vi "get matrix.vi"(8 "error in":errorcluster {"code" format="%.0x"}, 10 "Output Subunit":u32=1, 11 "Input Handle":cluster{"Session":u32, "Card number":u32}) -> (0 "error out":errorcluster, 1 "第二行":T1, 2 "第一行":T1, 3 "Output Handle":cluster{"Session":u32, "Card number":u32})   [LabVIEW 2018]
uses:
  ctl/matrix.ctl
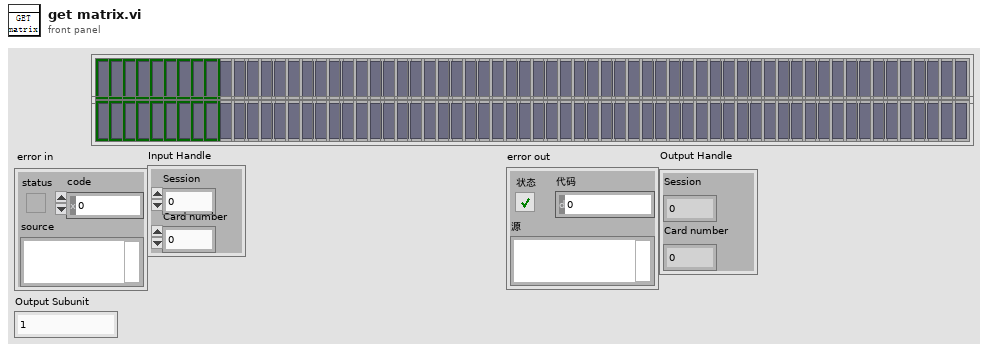
[diagram p1: front panel]
types:
  T1 = typedef "matrix.ctl" = cluster{"布尔":bool, "布尔 2":bool, "布尔 3":bool, "布尔 4":bool, "布尔 5":bool, "布尔 6":bool, "布尔 7":bool, "布尔 8":bool, "布尔 9":bool, "布尔 10":bool, "布尔 11":bool, "布尔 12":bool, "布尔 13":bool, "布尔 14":bool, "布尔 15":bool, "布尔 16":bool, "布尔 17":bool, "布尔 18":bool, "布尔 19":bool, "布尔 20":bool, "布尔 21":bool, "布尔 22":bool, "布尔 23":bool, "布尔 24":bool, "布尔 25":bool, "布尔 26":bool, "布尔 27":bool, "布尔 28":bool, "布尔 29":bool, "布尔 30":bool, "布尔 31":bool, "布尔 32":bool, "布尔 33":bool, "布尔 34":bool, "布尔 35":bool, "布尔 36":bool, "布尔 37":bool, "布尔 38":bool, "布尔 39":bool, "布尔 40":bool, "布尔 41":bool, "布尔 42":bool, "布尔 43":bool, "布尔 44":bool, "布尔 45":bool, "布尔 46":bool, "布尔 47":bool, "布尔 48":bool, "布尔 49":bool, "布尔 50":bool, "布尔 51":bool, "布尔 52":bool, "布尔 53":bool, "布尔 54":bool, "布尔 55":bool, "布尔 56":bool, "布尔 57":bool, "布尔 58":bool, "布尔 59":bool, "布尔 60":bool, "布尔 61":bool, "布尔 62":bool, "布尔 63":bool, "布尔 64":bool}
  T2 = cluster{"Boolean array[0]":bool, "Boolean array[1]":bool, "Boolean array[2]":bool, "Boolean array[3]":bool, "Boolean array[4]":bool, "Boolean array[5]":bool, "Boolean array[6]":bool, "Boolean array[7]":bool, "Boolean array[8]":bool, "Boolean array[9]":bool, "Boolean array[10]":bool, "Boolean array[11]":bool, "Boolean array[12]":bool, "Boolean array[13]":bool, "Boolean array[14]":bool, "Boolean array[15]":bool, "Boolean array[16]":bool, "Boolean array[17]":bool, "Boolean array[18]":bool, "Boolean array[19]":bool, "Boolean array[20]":bool, "Boolean array[21]":bool, "Boolean array[22]":bool, "Boolean array[23]":bool, "Boolean array[24]":bool, "Boolean array[25]":bool, "Boolean array[26]":bool, "Boolean array[27]":bool, "Boolean array[28]":bool, "Boolean array[29]":bool, "Boolean array[30]":bool, "Boolean array[31]":bool, "Boolean array[32]":bool, "Boolean array[33]":bool, "Boolean array[34]":bool, "Boolean array[35]":bool, "Boolean array[36]":bool, "Boolean array[37]":bool, "Boolean array[38]":bool, "Boolean array[39]":bool, "Boolean array[40]":bool, "Boolean array[41]":bool, "Boolean array[42]":bool, "Boolean array[43]":bool, "Boolean array[44]":bool, "Boolean array[45]":bool, "Boolean array[46]":bool, "Boolean array[47]":bool, "Boolean array[48]":bool, "Boolean array[49]":bool, "Boolean array[50]":bool, "Boolean array[51]":bool, "Boolean array[52]":bool, "Boolean array[53]":bool, "Boolean array[54]":bool, "Boolean array[55]":bool, "Boolean array[56]":bool, "Boolean array[57]":bool, "Boolean array[58]":bool, "Boolean array[59]":bool, "Boolean array[60]":bool, "Boolean array[61]":bool, "Boolean array[62]":bool, "Boolean array[63]":bool}
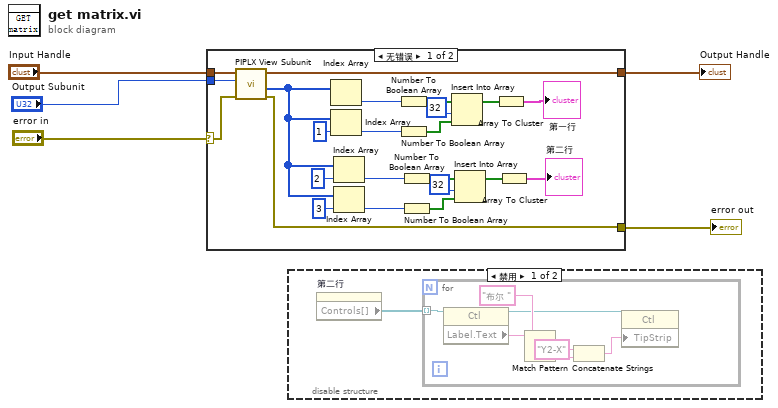
[diagram p0: block diagram]
diagram:
  n1 = case shown="无错误" "error in" {
    selector: "error in" -> [w6 w29]
    tunnel: "Input Handle" -> [w10 w30]
    tunnel: "Output Subunit" -> [w9 _]
    tunnel: [w8 w29] -> w2
    tunnel: [w7 w30] -> w1
    frame No Error {
      n2 = call <instrlib>:"PIPLX View Subunit.vi"("error in"=w6, "Output Subunit"=w9, "Input Handle"=w10) -> ("error out"=w8:errorcluster, "Data"=w12:u32[], "Output Handle"=w7:cluster{"Session":u32, "Card number":u32})  [unwired: 6 in]
      n3 = Index Array(array=w12) -> (element=w27:u32)  [unwired: 1 in]
      n4 = Index Array(array=w12, index=1 ("索引")) -> (element=w23:u32)
      n5 = Index Array(array=w12, index=2 ("索引")) -> (element=w14:u32)
      n6 = Index Array(array=w12, index=3 ("索引")) -> (element=w18:u32)
      n7 = Number To Boolean Array(number=w27) -> (Boolean array=w22:bool[])
      n8 = Number To Boolean Array(number=w23) -> (Boolean array=w26:bool[])
      n9 = Number To Boolean Array(number=w14) -> (Boolean array=w19:bool[])
      n10 = Number To Boolean Array(number=w18) -> (Boolean array=w15:bool[])
      n11 = Insert Into Array(array=w22, index=32 ("索引"), new element=w26) -> (w21:bool[])
      n12 = Insert Into Array(array=w19, index=32 ("索引"), new element=w15) -> (w20:bool[])
      n13 = Array To Cluster(array=w21) -> (cluster=→"第一行":T2)
      n14 = Array To Cluster(array=w20) -> (cluster=→"第二行":T2)
    }
    frame Error {
    }
  }
  "error out" <- w2
  "Output Handle" <- w1
  n15 = disable-structure shown="禁用" {
    frame Disabled {
      n16 = property on="第二行" class="Clust (严格)"() -> ("Controls[]"=w31:refnum<vi>[])  [unwired: 2 in, 2 out]
      n17 = for {
        tunnel: w31 -> [w38] mode=indexing
        n18 = property class="Ctl"(reference=w38) -> (reference out=w35:refnum<vi>, "Label.Text"=w37:string)  [unwired: 1 in, 1 out]
        n19 = Match Pattern(string=w37, regular expression="布尔 " ("正则表达式")) -> (after substring=w34:string)  [unwired: 1 in, 3 out]
        n20 = Concatenate Strings("Y2-X" ("字符串"), w34) -> (w32:string)
        n21 = property class="Ctl"(reference=w35, "TipStrip"=w32) -> ()  [unwired: 1 in, 2 out]
      }
    }
    frame Enabled {
    }
  }
